vi "S Parameter Measurement.vi"(8 "error in":errorcluster, 9 "RFmxVNA Settings":T2={"Resource Name"="VNA-5633", "vCal Name"="ni-cal1", "RFmxVNA Calset Enable"=FALSE, "RFmxVNA Calset Interpolation"=FALSE, "Calset File Path"="C:\\Users\\ies-pg-8881\\Desktop\\KB\\VNA 5633 CAL\\test1.ncst", "RFmxVNA attenuation mode"=enum."<None>", "RFmxVNA Port1 s2p file path"="C:\\Users\\ies-pg-8881\\Desktop\\KB\\VNA 5633 CAL\\260129_2SMA(F-F)_1-ps-cable0.3m.s2p", "RFmxVNA Port1 s-parameters orientation"=enum."Port1 Towards DUT", "RFmxVNA Port1 Power Compensation"=FALSE, "RFmxVNA Port2 s2p file path"="C:\\Users\\ies-pg-8881\\Desktop\\KB\\VNA 5633 CAL\\260129_2SMA(F-F)_1-ps-cable0.3m.s2p", "RFmxVNA Port2 s-parameters orientation"=enum."Port1 Towards DUT", "RFmxVNA Port2 Power Compensation"=FALSE, "Port1 Power Level (dBm)"=-10.0, "Port1 Test Receiver Attenuation (dB)"=0.0, "Port2 Power Level (dBm)"=-10.0, "Port2 Test Receiver Attenuation (dB)"=0.0, "IF Bandwidth (Hz)"=100000.0, "Frequency Sweep"={"Start Frequency (Hz)"=4000000000.0, "Stop Frequency (Hz)"=26500000000.0, "Number of Points"=200}} {"Frequency Sweep"."Stop Frequency (Hz)" format="%.3p"; "Frequency Sweep"."Start Frequency (Hz)" format="%.3p"; "IF Bandwidth (Hz)" format="%.2p"; "Port2 Test Receiver Attenuation (dB)" format="%.2f"; "Port2 Power Level (dBm)" format="%.2f"; "Port1 Test Receiver Attenuation (dB)" format="%.2f"; "Port1 Power Level (dBm)" format="%.2f"}, 11 "Test Configuration":T1={"Action"=enum."Calibrate", "Pulse Mode"={"Pulse Mode Enabled"=FALSE, "Pulse Period (s)"=0.001, "Pulse Modulator Delay (s)"=0.0, "Pulse Modulator Width (s)"=0.0001, "Pulse Acquisition Auto"=FALSE, "Pulse Acquisition Delay (s)"=2e-05, "Pulse Acquisition Width (s)"=4.665e-05}, "Frequency Sweep"={"Start Frequency (Hz)"=4000000000.0, "Stop Frequency (Hz)"=26500000000.0, "Number of Points"=200}, "S-Parameters"=["S11", "S12", "S21", "S22"], "Magnitude Units"=0, "Phase Trace Type"=0, "SnP File Path"="", "Averaging Enabled"=FALSE, "Averaging Count"=0} {"Phase Trace Type" items=["Wrapped", "Unwrapped"]; "Pulse Mode"."Pulse Acquisition Width (s)" format="%.2p"; "Pulse Mode"."Pulse Acquisition Delay (s)" format="%.2p"; "Pulse Mode"."Pulse Modulator Width (s)" format="%.2p"; "Pulse Mode"."Pulse Modulator Delay (s)" format="%.2p"; "Pulse Mode"."Pulse Period (s)" format="%.2p"; "Magnitude Units" items=["dB", "Linear"]; "Frequency Sweep"."Stop Frequency (Hz)" format="%.3p"; "Frequency Sweep"."Start Frequency (Hz)" format="%.3p"}) -> (0 "error out":errorcluster={"status"=TRUE, "code"=-1074134944, "source"="RFmxVNA Calibration Initiate.vi\r\n<ERR>IVI: (Hex 0xBFFA0060) Insufficient location information or resource not present in the system.  "}, 1 "VNA Status":string, 2 "S-Param Name":string[](array[string]), 3 "S-Param":dbl[][](array[numeric]), 5 "S-Param Phase":dbl[][](array[numeric]), 7 "S-Param Magnitude":dbl[][](array[numeric]))   [LabVIEW 2023]
uses:
  Controls/RFmxVNA Config - SParam.ctl
  Controls/Test Config - SParam.ctl
panel:
  out "Correction State":i32(ring) items=["None", "Corrected", "Interpolated", "Settings Modified"]
  out "SParam3":T3(graph)
  out "SParam1":T3(graph)
  out "SParam2":T3(graph)
  out "SParam0":T3(graph)
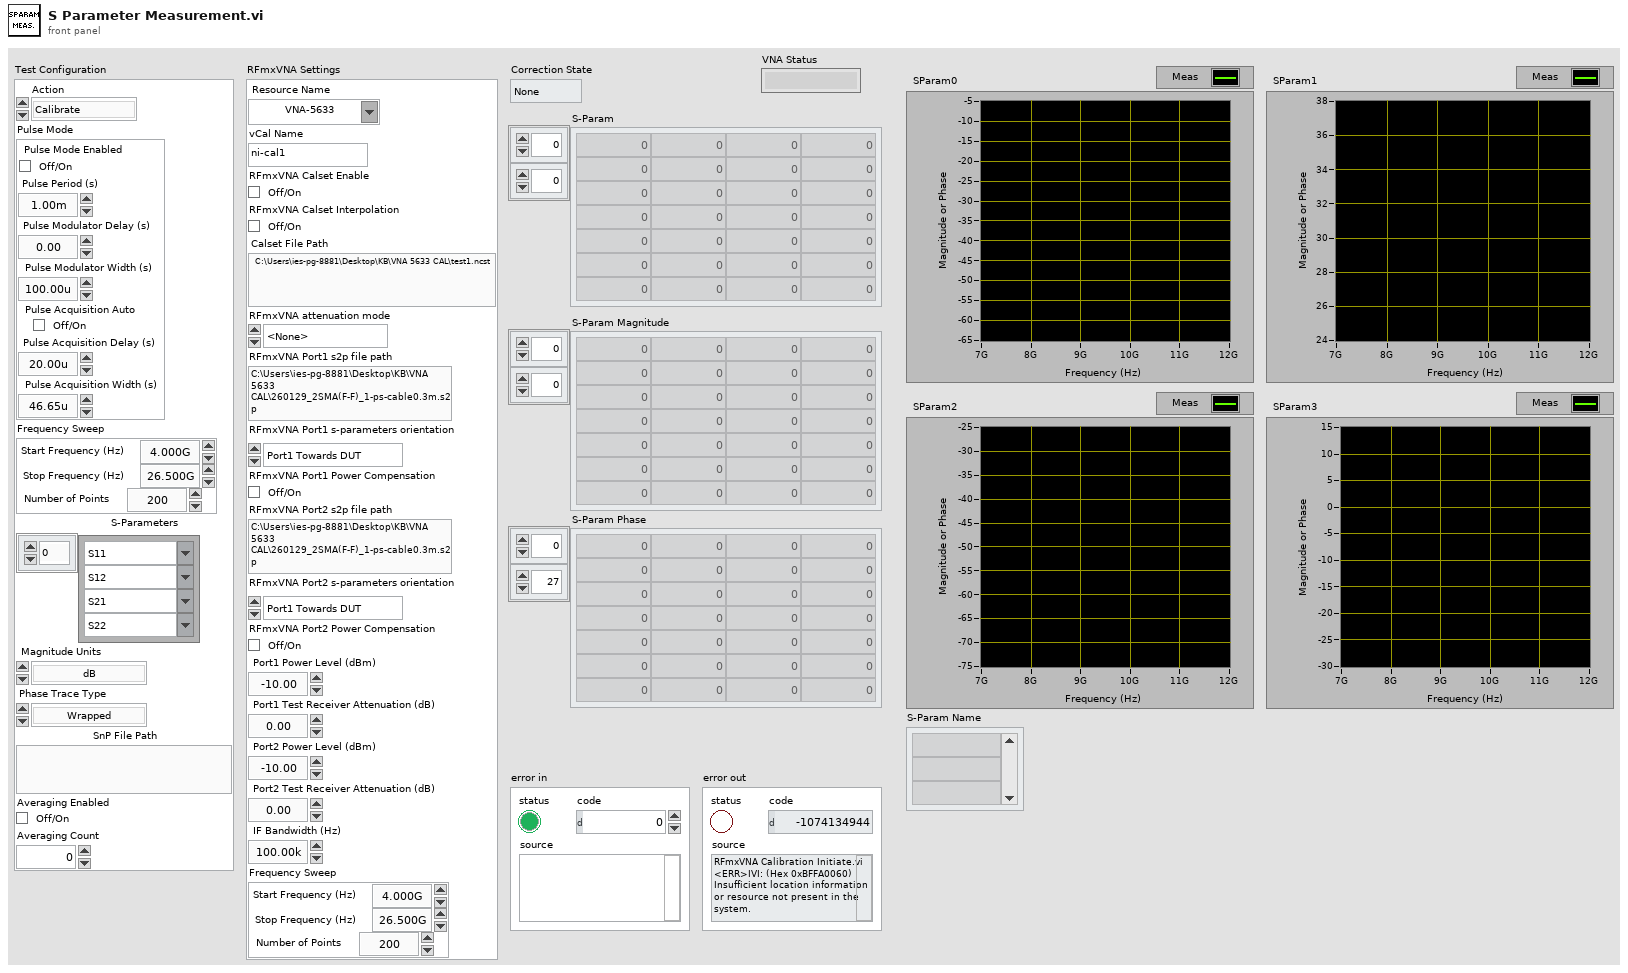
[diagram p1: front panel]
types:
  T1 = typedef "Test Config - SParam.ctl" = cluster{"Action":enum16{"Calibrate", "Measure"}, "Pulse Mode":cluster{"Pulse Mode Enabled":bool, "Pulse Period (s)":dbl, "Pulse Modulator Delay (s)":dbl, "Pulse Modulator Width (s)":dbl, "Pulse Acquisition Auto":bool, "Pulse Acquisition Delay (s)":dbl, "Pulse Acquisition Width (s)":dbl}, "Frequency Sweep":cluster{"Start Frequency (Hz)":dbl, "Stop Frequency (Hz)":dbl, "Number of Points":i32}, "S-Parameters":string[], "Magnitude Units":i32, "Phase Trace Type":i32, "SnP File Path":string, "Averaging Enabled":bool, "Averaging Count":u32}
  T2 = typedef "RFmxVNA Config - SParam.ctl" = cluster{"Resource Name":refnum<k15>, "vCal Name":string, "RFmxVNA Calset Enable":bool, "RFmxVNA Calset Interpolation":bool, "Calset File Path":string, "RFmxVNA attenuation mode":enum32{"<None>", "s2p File"}, "RFmxVNA Port1 s2p file path":string, "RFmxVNA Port1 s-parameters orientation":enum32{"Port1 Towards DUT", "Port2 Towards DUT"}, "RFmxVNA Port1 Power Compensation":bool, "RFmxVNA Port2 s2p file path":string, "RFmxVNA Port2 s-parameters orientation":enum32{"Port1 Towards DUT", "Port2 Towards DUT"}, "RFmxVNA Port2 Power Compensation":bool, "Port1 Power Level (dBm)":dbl, "Port1 Test Receiver Attenuation (dB)":dbl, "Port2 Power Level (dBm)":dbl, "Port2 Test Receiver Attenuation (dB)":dbl, "IF Bandwidth (Hz)":dbl, "Frequency Sweep":cluster{"Start Frequency (Hz)":dbl, "Stop Frequency (Hz)":dbl, "Number of Points":i32}}
  T3 = cluster{"Freq List (Hz)":dbl[], "Real Data":sgl[]}
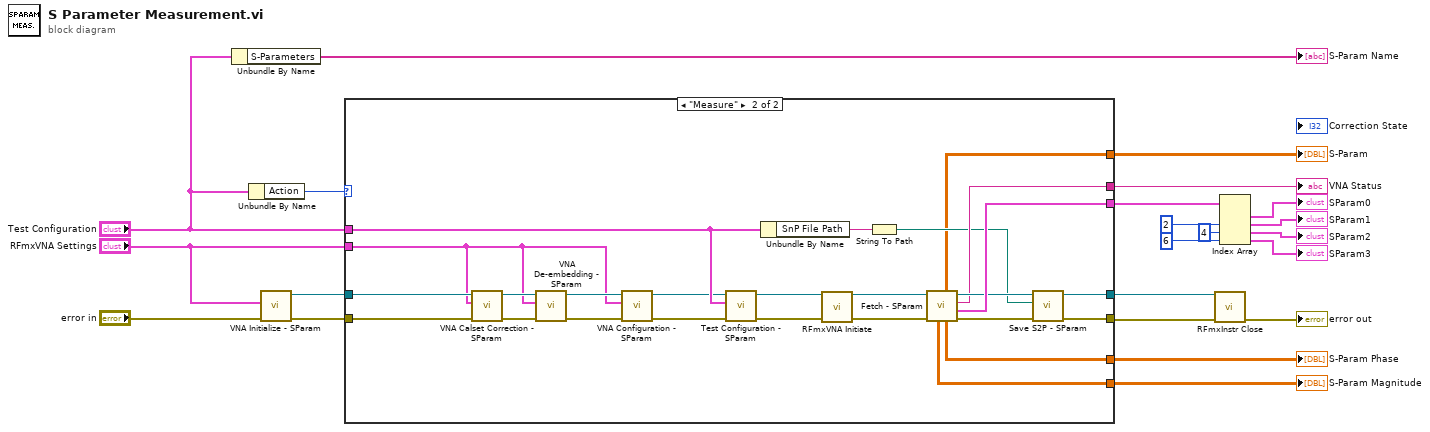
[diagram p0: block diagram]
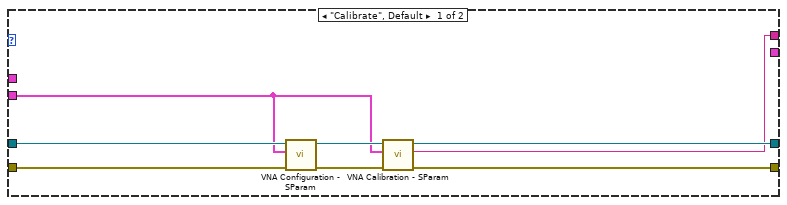
[diagram p2: hidden frame]
diagram:
  n1 = Unbundle By Name("Test Configuration") -> ("S-Parameters"=→"S-Param Name":string[])
  n2 = Unbundle By Name("Test Configuration") -> ("Action"=w9:enum16{"Calibrate", "Measure"})
  n3 = call "VNA Initialize - SParam.vi"("error in"="error in", "RFmxVNA Settings"="RFmxVNA Settings") -> ("error out"=w12:errorcluster, "RFmxVNA Session out"=w13:refnum<k21>)  [unwired: 8 in]
  n4 = case shown="\"Measure\"" w9 {
    tunnel: [_ w53] -> w22
    tunnel: [w30 w52] -> w19
    tunnel: [w29 w51] -> w18
    tunnel: [w28 w48] -> w3
    tunnel: w13 -> [w24 w36]
    tunnel: w12 -> [w25 w37]
    tunnel: "Test Configuration" -> [_ w47]
    tunnel: [_ w44] -> w11
    tunnel: "RFmxVNA Settings" -> [w23 w31]
    tunnel: [_ w41] -> w5
    tunnel: [_ w40] -> w4
    frame "Calibrate", Default {
      n5 = call "VNA Configuration - SParam.vi"("error in"=w25, "RFmxVNA Settings"=w23, "RFmxVNA Session in"=w24) -> ("error out"=w26:errorcluster, "RFmxVNA Session out"=w27:refnum<k21>)  [unwired: 7 in]
      n6 = call "VNA Calibration - SParam.vi"("error in"=w26, "RFmxVNA Settings"=w23, "RFmxVNA Session in"=w27) -> ("error out"=w29:errorcluster, "VNA Status"=w28:string, "RFmxVNA Session out"=w30:refnum<k21>)  [unwired: 6 in]
    }
    frame "Measure" {
      n7 = call "VNA Calset Correction - SParam.vi"("error in"=w37, "RFmxVNA Settings"=w31, "RFmxVNA Session in"=w36) -> ("error out"=w38:errorcluster, "RFmxVNA Session out"=w39:refnum<k21>)  [unwired: 7 in]
      n8 = call "VNA De-embedding - SParam.vi"("error in"=w38, "RFmxVNA Settings"=w31, "RFmxVNA Session in"=w39) -> ("error out"=w34:errorcluster, "RFmxVNA Session out"=w35:refnum<k21>)  [unwired: 7 in]
      n9 = call "VNA Configuration - SParam.vi"("error in"=w34, "RFmxVNA Settings"=w31, "RFmxVNA Session in"=w35) -> ("error out"=w32:errorcluster, "RFmxVNA Session out"=w33:refnum<k21>)  [unwired: 7 in]
      n10 = call "Test Configuration - SParam.vi"("error in"=w32, "Test Configuration"=w47, "RFmxVNA Session in"=w33) -> ("error out"=w42:errorcluster, "RFmxVNA Session out"=w43:refnum<k21>)  [unwired: 6 in, 1 out]
      n11 = Unbundle By Name(w47) -> ("SnP File Path"=w46:string)
      n12 = call <vilib>:"RFmxVNA Initiate.vi"("Instrument Handle In"=w43, "error in (no error)"=w42) -> ("Instrument Handle Out"=w55:refnum<k21>, "error out"=w54:errorcluster)  [unwired: 11 in, 1 out]
      n13 = String To Path(string=w46) -> (path=w45:path)
      n14 = call "Fetch - SParam.vi"("error in"=w54, "RFmxVNA Session in"=w55) -> ("error out"=w50:errorcluster, "Array"=w53:cluster{"X":dbl[], "Y1":sgl[]}[], "Status"=w48:string, "RFmxVNA Session out"=w49:refnum<k21>, "S-Param Phase"=w40:dbl[][], "S-Param"=w44:dbl[][], "S-Param Magnitude"=w41:dbl[][])  [unwired: 3 in]
      n15 = call "Save S2P - SParam.vi"("error in"=w50, "SnP File Path"=w45, "Refnum in"=w49) -> ("error out"=w51:errorcluster, "Refnum out"=w52:refnum<k21>)  [unwired: 7 in]
    }
  }
  "S-Param" <- w11
  "S-Param Magnitude" <- w5
  "S-Param Phase" <- w4
  "VNA Status" <- w3
  n16 = call <vilib>:"RFmxInstr Close.vi"("Instrument Handle In"=w19, "error in (no error)"=w18) -> ("error out"=→"error out":errorcluster)  [unwired: 13 in]
  n17 = Index Array(array=w22, index #2=2 ("index"), index #3=4 ("index"), index #4=6 ("index")) -> (element #1=→"SParam0":cluster{"X":dbl[], "Y1":sgl[]}, element #2=→"SParam1":cluster{"X":dbl[], "Y1":sgl[]}, element #3=→"SParam2":cluster{"X":dbl[], "Y1":sgl[]}, element #4=→"SParam3":cluster{"X":dbl[], "Y1":sgl[]})  [unwired: 1 in]
